vi "I Term.vi"(7 "Output Range":T1={"Min"=-50.0, "Max"=50.0}, 8 "Error":dbl, 9 "I Gain":dbl=0.5, 10 "Last Sum":dbl=100.0, 11 "dT":dbl=0.1) -> (1 "Output":dbl, 2 "Sum":dbl, 5 "Remaining Range":T1)   [LabVIEW 2020, in "IG PID.lvlib" / "PID.lvclass"]
uses:
  PID.lvclass
  Output Range.ctl
  IG PID.lvlib
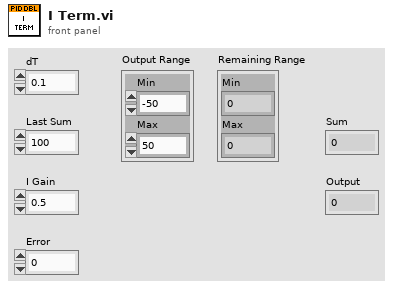
[diagram p1: front panel]
types:
  T1 = typedef "IG PID.lvlib/Output Range.ctl" = cluster{"Min":dbl, "Max":dbl}
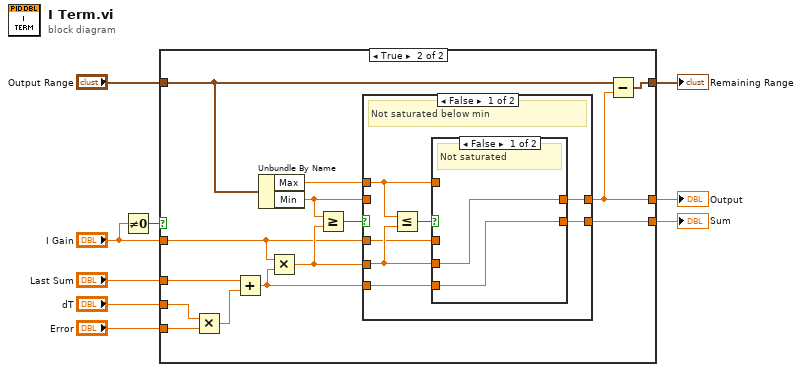
[diagram p0: block diagram]
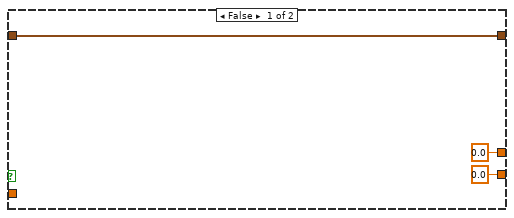
[diagram p2: hidden frame]
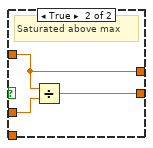
[diagram p3: hidden frame]
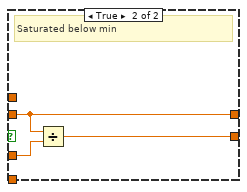
[diagram p4: hidden frame]
diagram:
  n1 = Not Equal To 0?(x="I Gain") -> (x != 0?=w1:bool)
  n2 = case shown="True" w1 {
    tunnel: "Error" -> [_ w26]
    tunnel: "dT" -> [_ w25]
    tunnel: "Last Sum" -> [_ w24]
    tunnel: [0.0 w18] -> w6
    tunnel: "Output Range" -> [w12 w17]
    tunnel: [0.0 ("Min") w16] -> w4
    tunnel: [w12 w15] -> w3
    tunnel: "I Gain" -> [_ w13]
    frame False {
    }
    frame True {
      n3 = Multiply(x=w25, y=w26) -> (x*y=w23:dbl)
      n4 = Add(x=w24, y=w23) -> (x+y=w14:dbl)
      n5 = Unbundle By Name(w17) -> ("Max"=w19:dbl, "Min"=w20:dbl)
      n6 = Multiply(x=w13, y=w14) -> (x*y=w21:dbl)
      n7 = Greater Or Equal?(x=w20, y=w21) -> (x >= y?=w22:bool)
      n8 = case shown="False" w22 {
        tunnel: w21 -> [w31 _]
        tunnel: w13 -> [w30 w41]
        tunnel: w20 -> [_ w39]
        tunnel: w19 -> [w32 _]
        tunnel: [w29 w40] -> w18
        tunnel: [w28 w39] -> w16
        tunnel: w14 -> [w27 _]
        frame False {
          # "Not saturated below min"
          n9 = Less Or Equal?(x=w32, y=w31) -> (x <= y?=w33:bool)
          n10 = case shown="False" w33 {
            tunnel: w32 -> [_ w36]
            tunnel: w31 -> [w34 _]
            tunnel: w30 -> [_ w38]
            tunnel: [w35 w37] -> w29
            tunnel: [w34 w36] -> w28
            tunnel: w27 -> [w35 _]
            frame False {
              # "Not saturated"
            }
            frame True {
              # "Saturated above max"
              n11 = Divide(x=w36, y=w38) -> (x/y=w37:dbl)
            }
          }
        }
        frame True {
          # "Saturated below min"
          n12 = Divide(x=w39, y=w41) -> (x/y=w40:dbl)
        }
      }
      n13 = Subtract(x=w17, y=w16) -> (x-y=w15:T1)
    }
  }
  "Remaining Range" <- w3
  "Output" <- w4
  "Sum" <- w6
